vi "Read MDA.vi"(8 "error in (no error)":errorcluster, 11 "Airmar Data in":refnum<class "Airmar Data.lvclass">) -> (0 "error out":errorcluster, 2 "MDA":T1, 3 "Airmar Data out":refnum<class "Airmar Data.lvclass">)   [LabVIEW 2013, in "Airmar Data.lvclass"]
uses:
  Airmar Data.lvclass
  Airmar Data.lvclass/Airmar Data.ctl
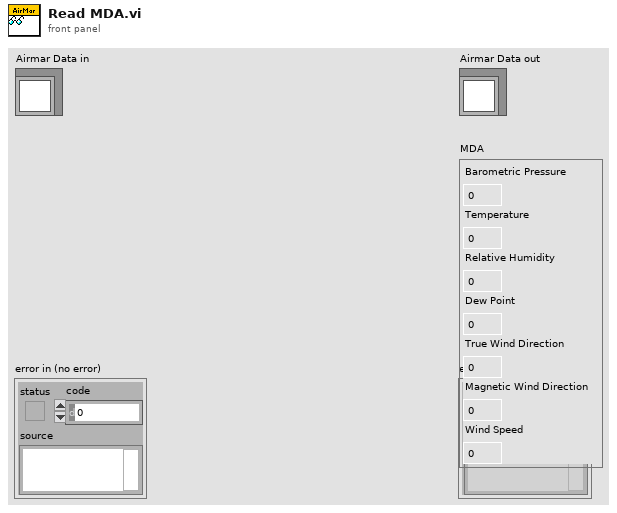
[diagram p1: front panel]
types:
  T1 = cluster{"Barometric Pressure":dbl, "Temperature":dbl, "Relative Humidity":dbl, "Dew Point":dbl, "True Wind Direction":dbl, "Magnetic Wind Direction":dbl, "Wind Speed":dbl}
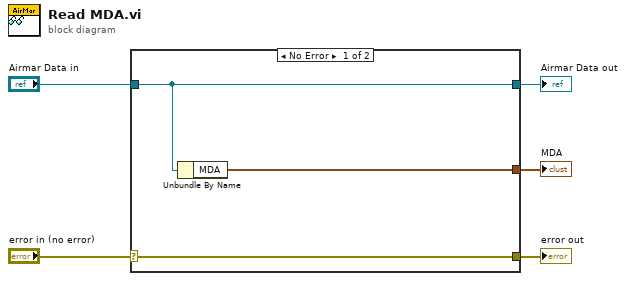
[diagram p0: block diagram]
diagram:
  n1 = case shown="No Error" "error in (no error)" {
    selector: "error in (no error)" -> [w8 w9]
    tunnel: [w8 w9] -> w4
    tunnel: [w7 w10] -> w2
    tunnel: "Airmar Data in" -> [w7 w10]
    tunnel: [w6 _] -> w1
    frame No Error {
      n2 = Unbundle By Name(w7) -> ("MDA"=w6:T1)
    }
    frame Error {
    }
  }
  "error out" <- w4
  "Airmar Data out" <- w2
  "MDA" <- w1
